vi "Check.vi"() -> ()   [LabVIEW 2019]
uses:
  Z_Hswitch_little.xctl
  Y_source.ctl
  Counter/Counter.lvlib
  Logik/Logik.lvlib
  Heating.lvlib
panel:
  out "Boolean":bool
  in  "Z_Source":T1
  in  "connect":bool
  in  "Z_Hswitch":bool(xcontrol)
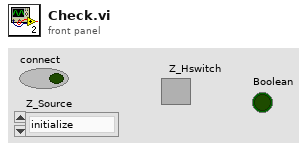
[diagram p1: front panel]
types:
  T1 = typedef "Heating.lvlib/Y_source.ctl" = enum8{"initialize", "local disabled", "local hand", "hand", "auto", "dist"}
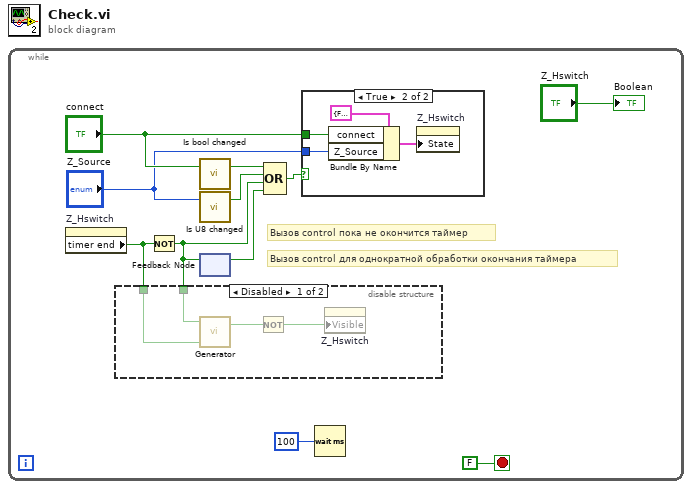
[diagram p0: block diagram]
diagram:
  n1 = while {
    stop <- FALSE stop-if-true
    # "Вызов control пока не окончится таймер"
    # "Вызов control для однократной обработки окончания таймера"
    n2 = property on="Z_Hswitch" class="Z_Hswitch_little (strict)"() -> ("timer end"=w3:bool)  [unwired: 2 in, 2 out]
    n3 = Not(x=w3) -> (.not. x?=w1:bool)
    n4 = disable-structure shown="Disabled" {
      disable-tunnel: w3 -> [w13 _]
      disable-tunnel: w1 -> [w12 _]
      frame Disabled {
        n5 = call "Generator.vi"("R"=w13, "ON (F)"=w12) -> ("Q"=w14:bool)  [unwired: 2 in]
        n6 = Not(x=w14) -> (.not. x?=w15:bool)
        n7 = property on="Z_Hswitch" class="Z_Hswitch_little (strict)"("Visible"=w15) -> ()  [unwired: 2 in, 2 out]
      }
      frame Enabled {
      }
    }
    n8 = call "Is bool changed.vi"("in"="connect") -> ("changed or first call?"=w6:bool)  [unwired: 2 in]
    n9 = call "Is U8 changed.vi"("in"="Z_Source") -> ("changed or first call?"=w7:bool)  [unwired: 2 in]
    n10 = feedback-in #1(w1) -> ()
    n11 = feedback #1() -> (w2:bool)  [unwired: 1 in]
    n12 = Compound Arithmetic op=OR(w6, w7, w1, w2) -> (w9:bool)
    n13 = case shown="True" w9 {
      tunnel: "connect" -> [_ w18]
      tunnel: "Z_Source" -> [_ w17]
      frame False {
      }
      frame True {
        n14 = Bundle By Name(cluster=cluster{"connect":bool, "Z_Source":T1} {"connect"=FALSE, "Z_Source"=enum."initialize"} ("source"), "connect"=w18, "Z_Source"=w17) -> (w16:cluster{"connect":bool, "Z_Source":T1})
        n15 = property on="Z_Hswitch" class="Z_Hswitch_little (strict)"("State"=w16) -> ()  [unwired: 2 in, 2 out]
      }
    }
    n16 = Wait (ms)(milliseconds to wait=u32 100) -> ()  [unwired: 1 out]
    "Boolean" <- "Z_Hswitch"
  }
